vi "Get X Array dx.vi"(8 "error in (no error)":errorcluster, 11 "XY-data":cluster{"X-array":dbl[], "Y-array":dbl[]}) -> (0 "error out":errorcluster, 1 "X0":dbl, 2 "dX":dbl, 3 "XY-data out":cluster{"X-array":dbl[], "Y-array":dbl[]})   [LabVIEW 2016, in "xy_utilities.lvlib"]
uses:
  xy_utilities.lvlib
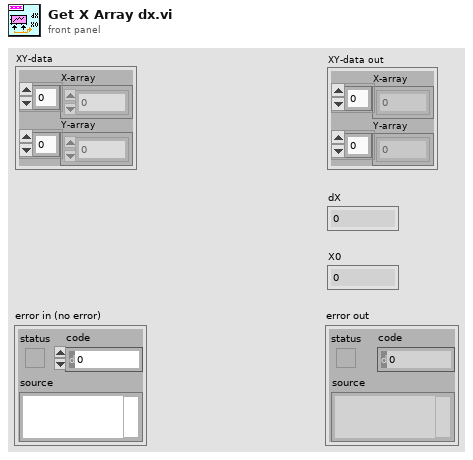
[diagram p1: front panel]
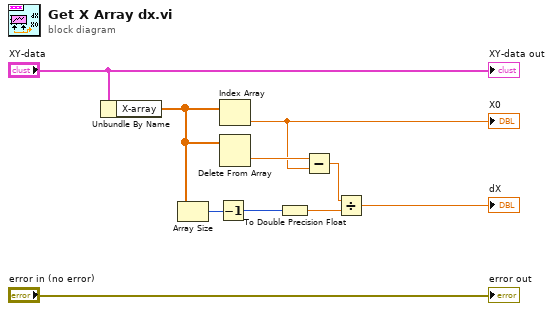
[diagram p0: block diagram]
diagram:
  n1 = Unbundle By Name("XY-data") -> ("X-array"=w5:dbl[])
  n2 = Array Size(array=w5) -> (size(s)=w10:i32)
  n3 = Decrement(x=w10) -> (x-1=w2:i32)
  n4 = Index Array(array=w5) -> (element=w3:dbl)  [unwired: 1 in]
  "X0" <- w3
  n5 = Delete From Array(array=w5) -> (deleted portion=w4:dbl)  [unwired: 2 in, 1 out]
  n6 = To Double Precision Float(number=w2) -> (double precision float=w9:dbl)
  n7 = Subtract(x=w4, y=w3) -> (x-y=w1:dbl)
  n8 = Divide(x=w1, y=w9) -> (x/y=→"dX":dbl)
  "error out" <- "error in (no error)"
  "XY-data out" <- "XY-data"
